vi "translate and offset.vi"(0 "robot location":cluster{"x":i32, "y":i32, "direction":dbl}, 1 "rect":T1) -> (2 "index 0":i32, 3 "length 0":i32, 4 "index 1":i32, 5 "length 1":i32)   [LabVIEW 2009]
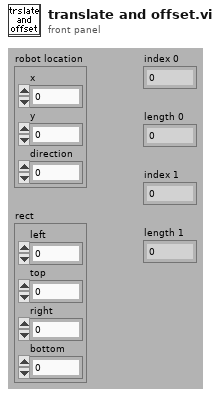
[diagram p1: front panel]
types:
  T1 = cluster{"left":i16, "top":i16, "right":i16, "bottom":i16}
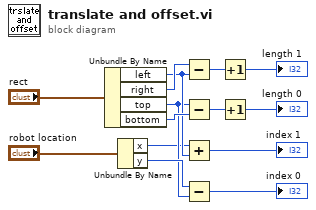
[diagram p0: block diagram]
diagram:
  n1 = Unbundle By Name("rect") -> ("left"=w10:i16, "right"=w11:i16, "top"=w4:i16, "bottom"=w12:i16)
  n2 = Unbundle By Name("robot location") -> ("x"=w1:i32, "y"=w5:i32)
  n3 = Subtract(x=w11, y=w10) -> (x-y=w9:i16)
  n4 = Subtract(x=w4, y=w12) -> (x-y=w8:i16)
  n5 = Add(x=w1, y=w10) -> (x+y=→"index 1":i32)
  n6 = Subtract(x=w5, y=w4) -> (x-y=→"index 0":i32)
  n7 = Increment(x=w9) -> (x+1=→"length 1":i16)
  n8 = Increment(x=w8) -> (x+1=→"length 0":i16)
